vi "3feladat.vi"() -> ()   [LabVIEW 2015]
panel:
  out "Boolean":bool
  out "Meter":dbl(knob) scale=1.0..6.0
  out "Numeric":dbl
  in  "OK Button":bool
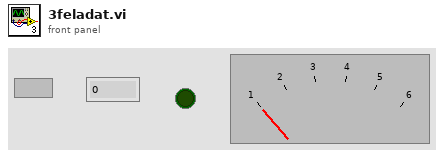
[diagram p1: front panel]
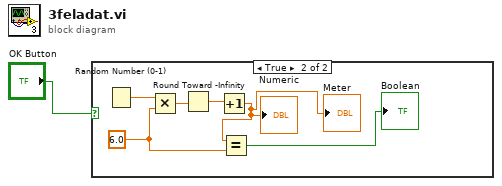
[diagram p0: block diagram]
diagram:
  n1 = case shown="True" "OK Button" {
    frame False {
    }
    frame True {
      w3 = 6.0
      n2 = Random Number (0-1)() -> (number: 0 to 1=w7:dbl)
      n3 = Multiply(x=w7, y=w3) -> (x*y=w6:dbl)
      n4 = Round Toward -Infinity(1:w6) -> (0:w5:dbl)
      n5 = Increment(x=w5) -> (x+1=w4:dbl)
      "Numeric" <- w4
      "Meter" <- w4
      n6 = Equal?(x=w4, y=w3) -> (x = y?=→"Boolean":bool)
    }
  }
